vi "DatabaseMain.vi"() -> ()   [LabVIEW 2019]
uses:
  ProductsCluster.ctl
  ProgramStates.ctl
  ProductsDataToWork.ctl
  SortWork.ctl
  <vilib>/Utility/file.llb/Read Delimited Spreadsheet (string).vi
panel:
  in  "?":bool
  in  "?":bool
  in  "?":bool
  in  "?":bool
  in  "?":bool
  in  "?":bool
  in  "?":bool
  in  "Search Value":string
  in  "SearchBy":enum16{"Name", "Number", "Producer"}(ring)=enum."Number"
  in  "?":bool
  in  "?":bool
  in  "?":bool
  in  "?":bool
  out "?":T1={"Numer Produktu"="1112", "Nazwa Produktu"="Laptop", "Wytwórca"="Dell"}
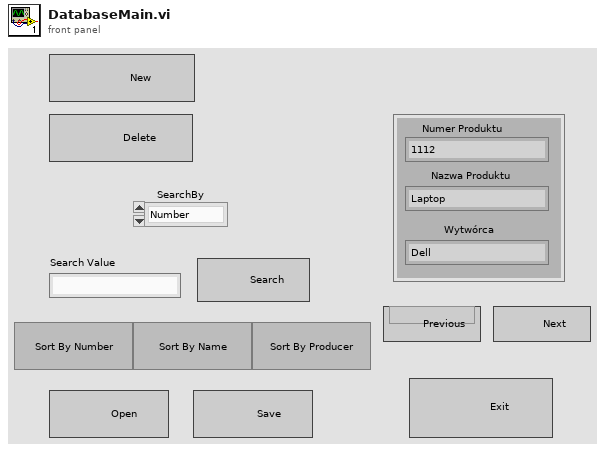
[diagram p1: front panel]
types:
  T1 = typedef "ProductsCluster.ctl" = cluster{"Numer Produktu":string, "Nazwa Produktu":string, "Wytwórca":string}
  T2 = typedef "ProductsDataToWork.ctl" = cluster{"Products":T1[], "CurrentProduct":i32, "SearchBy":enum16{"Name", "Number", "Producer"}, "SearchValue":string, "DataFilePath":path, "SortBy":enum32{"Name", "Number", "Producer"}}
  T3 = typedef "ProgramStates.ctl" = enum16{"Init", "Idle", "Open", "ShowPrevorious", "ShowNext", "Search", "SortByName", "SortByProducer", "SortByNumber", "Sort", "Add", "Delete", "Save", "Exit"}
  T4 = typedef "SortWork.ctl" = enum32{"Name", "Number", "Producer"}
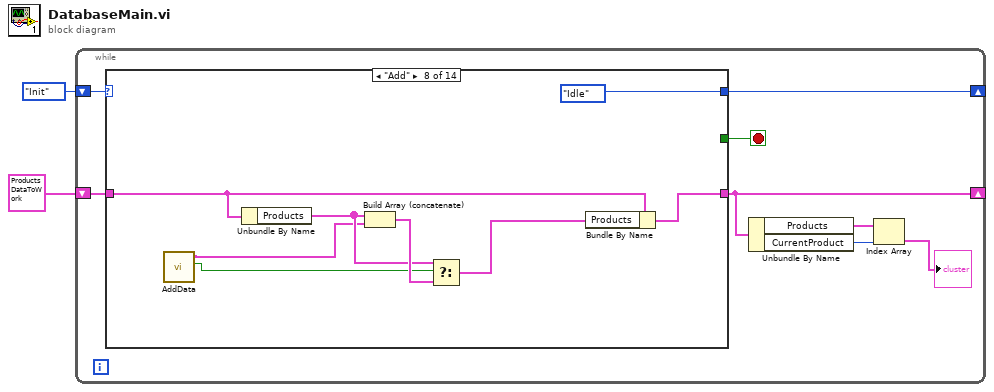
[diagram p0: block diagram]
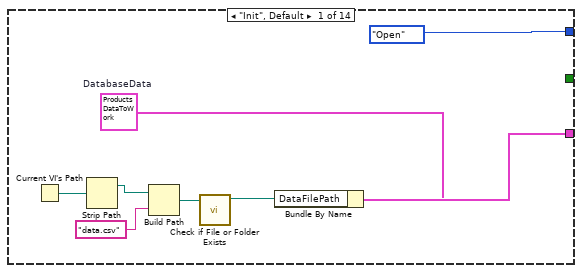
[diagram p2: hidden frame]
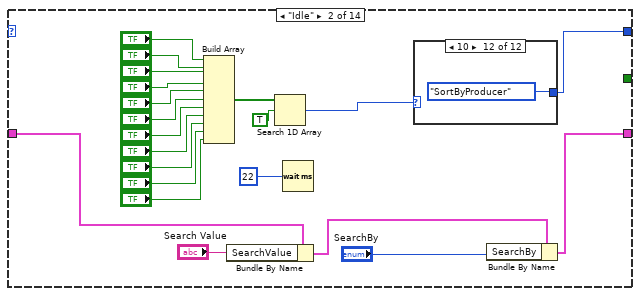
[diagram p3: hidden frame]
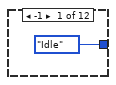
[diagram p4: hidden frame]
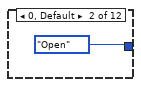
[diagram p5: hidden frame]
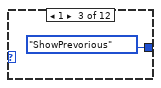
[diagram p6: hidden frame]
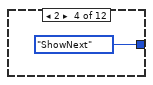
[diagram p7: hidden frame]
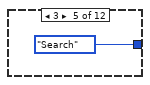
[diagram p8: hidden frame]
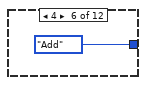
[diagram p9: hidden frame]
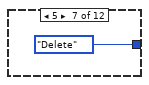
[diagram p10: hidden frame]
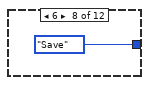
[diagram p11: hidden frame]
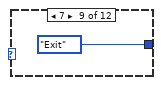
[diagram p12: hidden frame]
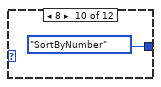
[diagram p13: hidden frame]
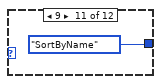
[diagram p14: hidden frame]
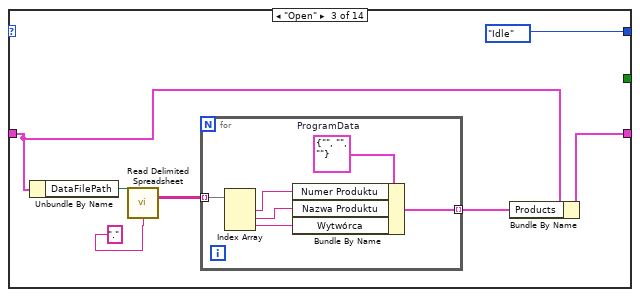
[diagram p15: hidden frame]
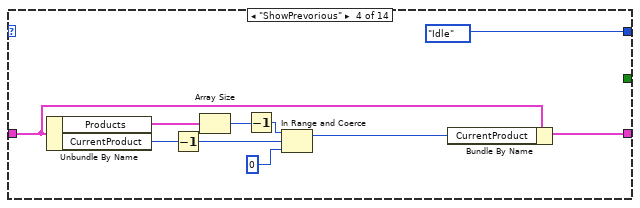
[diagram p16: hidden frame]
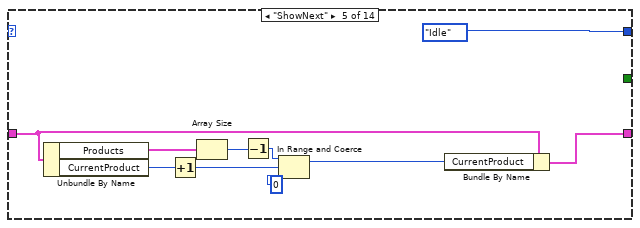
[diagram p17: hidden frame]
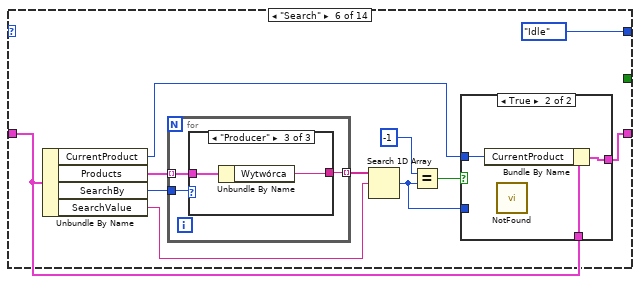
[diagram p18: hidden frame]
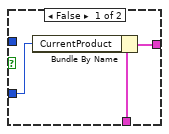
[diagram p19: hidden frame]
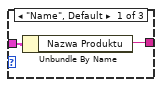
[diagram p20: hidden frame]
diagram:
  n1 = while {
    shift-right: [w5] -> _
    shift-left: T2 {"Products"=[], "CurrentProduct"=0, "SearchBy"=enum."Name", "SearchValue"="", "DataFilePath"=path "", "SortBy"=enum."Name"} ("DatabaseData") -> [w4]
    shift-right: [w7] -> _
    shift-left: ProgramStates."Init" -> [w6]
    stop <- w3 stop-if-true
    n2 = case shown="\"Add\"" w6 {
      tunnel: [ProgramStates."Open" w25 ProgramStates."Idle" ProgramStates."Idle" ProgramStates."Idle" ProgramStates."Idle" ProgramStates."Idle" ProgramStates."Idle" ProgramStates."Idle" ProgramStates."Idle" ProgramStates."Exit" ProgramStates."Sort" ProgramStates."Sort" ProgramStates."Sort"] -> w7
      tunnel: [w18 w27 w58 w66 w76 w87 w116 w119 w129 w145 T2 {"Products"=[], "CurrentProduct"=0, "SearchBy"=enum."Name", "SearchValue"="", "DataFilePath"=path "", "SortBy"=enum."Name"} ("DatabaseData") w153 w157 w161] -> w5
      tunnel: w4 -> [_ w19 w52 w67 w77 w89 w113 w120 w130 w145 w149 w154 w156 w160]
      tunnel: [_ _ _ _ _ _ _ _ _ _ TRUE _ _ _] -> w3
      frame "Init", Default {
        w16 = T2 {"Products"=[], "CurrentProduct"=0, "SearchBy"=enum."Name", "SearchValue"="", "DataFilePath"=path "", "SortBy"=enum."Name"}  # DatabaseData
        n3 = Current VI's Path() -> (path=w11:path)
        n4 = Strip Path(path=w11) -> (stripped path=w12:path)  [unwired: 1 out]
        n5 = Build Path(base path=w12, name or relative path="data.csv") -> (appended path=w14:path)
        n6 = call <vilib>:"Check if File or Folder Exists.vi"("path"=w14) -> ("dup path"=w13:path)  [unwired: 8 in, 2 out]
        n7 = Bundle By Name(cluster=w16, "DataFilePath"=w13) -> (w18:T2)
      }
      frame "Idle" {
        n8 = Build Array("?", "?", "?", "?", "?", "?", "?", "?", "?", "?", "?") -> (w31:bool[])
        n9 = Bundle By Name(cluster=w19, "SearchValue"="Search Value") -> (w23:T2)
        n10 = Search 1D Array(1D array=w31, element=TRUE) -> (index of element=w30:i32)  [unwired: 1 in]
        n11 = Wait (ms)(milliseconds to wait=u32 22) -> ()  [unwired: 1 out]
        n12 = case shown="10" w30 {
          tunnel: [ProgramStates."Idle" ProgramStates."Open" ProgramStates."ShowPrevorious" ProgramStates."ShowNext" ProgramStates."Search" ProgramStates."Add" ProgramStates."Delete" ProgramStates."Save" ProgramStates."Exit" ProgramStates."SortByNumber" ProgramStates."SortByName" ProgramStates."SortByProducer"] -> w25
          frame -1 {
          }
          frame 0, Default {
          }
          frame 1 {
          }
          frame 2 {
          }
          frame 3 {
          }
          frame 4 {
          }
          frame 5 {
          }
          frame 6 {
          }
          frame 7 {
          }
          frame 8 {
          }
          frame 9 {
          }
          frame 10 {
          }
        }
        n13 = Bundle By Name(cluster=w23, "SearchBy"="SearchBy") -> (w27:T2)
      }
      frame "Open" {
        n14 = Unbundle By Name(w52) -> ("DataFilePath"=w56:path)
        n15 = call-poly <vilib>:"Read Delimited Spreadsheet.vi"("file path (dialog if empty)"=w56, "delimiter (\\t)"=".") -> ("all rows"=w54:string[][])  [unwired: 8 in, 5 out]
        n16 = for {
          tunnel: w54 -> [w64] mode=indexing
          tunnel: [w60] -> w53 mode=indexing
          w59 = T1 {"Numer Produktu"="", "Nazwa Produktu"="", "Wytwórca"=""}  # ProgramData
          n17 = Index Array(array=w64) -> (element #1=w63:string, element #2=w62:string, element #3=w61:string)  [unwired: 3 in]
          n18 = Bundle By Name(cluster=w59, "Numer Produktu"=w63, "Nazwa Produktu"=w62, "Wytwórca"=w61) -> (w60:T1)
        }
        n19 = Bundle By Name(cluster=w52, "Products"=w53) -> (w58:T2)
      }
      frame "ShowPrevorious" {
        n20 = Unbundle By Name(w67) -> ("Products"=w70:T1[], "CurrentProduct"=w69:i32)
        n21 = Decrement(x=w69) -> (x-1=w71:i32)
        n22 = Array Size(array=w70) -> (size(s)=w72:i32)
        n23 = Decrement(x=w72) -> (x-1=w73:i32)
        n24 = In Range and Coerce(upper limit=w73, x=w71, lower limit=0) -> (coerced(x)=w74:i32)  [unwired: 1 out]
        n25 = Bundle By Name(cluster=w67, "CurrentProduct"=w74) -> (w66:T2)
      }
      frame "ShowNext" {
        n26 = Unbundle By Name(w77) -> ("Products"=w80:T1[], "CurrentProduct"=w79:i32)
        n27 = Increment(x=w79) -> (x+1=w81:i32)
        n28 = Array Size(array=w80) -> (size(s)=w82:i32)
        n29 = Decrement(x=w82) -> (x-1=w83:i32)
        n30 = In Range and Coerce(upper limit=w83, x=w81, lower limit=0) -> (coerced(x)=w84:i32)  [unwired: 1 out]
        n31 = Bundle By Name(cluster=w77, "CurrentProduct"=w84) -> (w76:T2)
      }
      frame "Search" {
        n32 = Unbundle By Name(w89) -> ("CurrentProduct"=w88:i32, "Products"=w95:T1[], "SearchBy"=w93:enum16{"Name", "Number", "Producer"}, "SearchValue"=w92:string)
        n33 = for {
          tunnel: w95 -> [w104] mode=indexing
          tunnel: [w103] -> w94 mode=indexing
          tunnel: w93 -> [w102]
          n34 = case shown="\"Producer\"" w102 {
            tunnel: w104 -> [w105 w108 w110]
            tunnel: [w106 w107 w109] -> w103
            frame "Name", Default {
              n35 = Unbundle By Name(w105) -> ("Nazwa Produktu"=w106:string)
            }
            frame "Number" {
              n36 = Unbundle By Name(w108) -> ("Numer Produktu"=w107:string)
            }
            frame "Producer" {
              n37 = Unbundle By Name(w110) -> ("Wytwórca"=w109:string)
            }
          }
        }
        n38 = Search 1D Array(1D array=w94, element=w92) -> (index of element=w85:i32)  [unwired: 1 in]
        n39 = Equal?(x=-1 ("y"), y=w85) -> (x = y?=w91:bool)
        n40 = case shown="True" w91 {
          tunnel: w89 -> [w98 w101]
          tunnel: w88 -> [_ w100]
          tunnel: [w96 w99] -> w87
          tunnel: w85 -> [w97 _]
          frame False {
            n41 = Bundle By Name(cluster=w98, "CurrentProduct"=w97) -> (w96:T2)
          }
          frame True {
            n42 = Bundle By Name(cluster=w101, "CurrentProduct"=w100) -> (w99:T2)
            n43 = call "NotFound.vi"() -> ()  [unwired: 12 in]
          }
        }
      }
      frame "Sort" {
        n44 = Unbundle By Name(w113) -> ("Products"=w115:T1[])
        n45 = Unbundle By Name(w113) -> ("SortBy"=w112:enum32{"Name", "Number", "Producer"})
        n46 = call "SortData.vi"("SortBy"=w112, "ProductsToSort"=w115) -> ("ProductsSorted"=w114:T1[])  [unwired: 9 in]
        n47 = Bundle By Name(cluster=w113, "Products"=w114) -> (w116:T2)
        n48 = call "SortOk.vi"() -> ()  [unwired: 12 in]
      }
      frame "Add" {
        n49 = call "AddData.vi"() -> (2:w117:bool, "ProgramData 2"=w118:T1)  [unwired: 10 in]
        n50 = Unbundle By Name(w120) -> ("Products"=w121:T1[])
        n51 = Build Array (concatenate)(w121, w118) -> (w122:T1[])
        n52 = Select(t=w121, s=w117, f=w122) -> (s? t:f=w123:T1[])
        n53 = Bundle By Name(cluster=w120, "Products"=w123) -> (w119:T2)
      }
      frame "Delete" {
        n54 = Unbundle By Name(w130) -> ("Products"=w128:T1[], "CurrentProduct"=w127:i32)
        n55 = Delete From Array(array=w128, index=w127) -> (deleted portion=w126:T1, array with subset deleted=w125:T1[])  [unwired: 1 in]
        n56 = call "DeletedCommunity.vi"("ProgramData"=w126) -> ("ReturnedStates"=w131:enum16{"DeleteConfirmed", "CancelDelete"})  [unwired: 10 in]
        n57 = case shown="\"DeleteConfirmed\", Default" w131 {
          tunnel: w130 -> [w134 w141]
          tunnel: [w135 w140] -> w129
          tunnel: w128 -> [_ w139]
          tunnel: w127 -> [w137 w138]
          tunnel: w125 -> [w133 _]
          frame "DeleteConfirmed", Default {
            n58 = call "CurrentValue.vi"("CurrentIn"=w137) -> ("CurrentOut"=w136:i32)  [unwired: 10 in]
            n59 = Bundle By Name(cluster=w134, "Products"=w133, "CurrentProduct"=w136) -> (w135:T2)
          }
          frame "CancelDelete" {
            n60 = Bundle By Name(cluster=w141, "Products"=w139, "CurrentProduct"=w138) -> (w140:T2)
          }
        }
      }
      frame "Save" {
        n61 = Unbundle By Name(w145) -> ("Products"=w143:T1[], "DataFilePath"=w142:path)
        n62 = call "SaveData.vi"("DataFilePath"=w142, "Products"=w143) -> ()  [unwired: 10 in]
        n63 = call "SaveOk.vi"() -> ()  [unwired: 12 in]
      }
      frame "Exit" {
        n64 = Unbundle By Name(w149) -> ("Products"=w148:T1[], "DataFilePath"=w147:path)
        n65 = call "SaveData.vi"("DataFilePath"=w147, "Products"=w148) -> ()  [unwired: 10 in]
      }
      frame "SortByName" {
        n66 = Bundle By Name(cluster=w154, "SortBy"=SortWork."Name") -> (w153:T2)
      }
      frame "SortByProducer" {
        n67 = Bundle By Name(cluster=w156, "SortBy"=SortWork."Producer") -> (w157:T2)
      }
      frame "SortByNumber" {
        n68 = Bundle By Name(cluster=w160, "SortBy"=SortWork."Number") -> (w161:T2)
      }
    }
    n69 = Unbundle By Name(w5) -> ("Products"=w9:T1[], "CurrentProduct"=w10:i32)
    n70 = Index Array(array=w9, index=w10) -> (element=→"?":T1)
  }
